vi "IMAQDevice.destructor.vi"(0 "i ref in":refnum<vi>, 5 "error in (no error)":errorcluster) -> (19 "error out":errorcluster)   [LabVIEW 2014, in "IMAQDevice.lvlib"]
doc: "This is the destructor of a class.\n\nLicense Agreement for this software:\n\nCopyright (C)\nGesellschaft für Schwerionenforschung, GSI\nPlanckstr. 1\n64291 Darmstadt\nGermany\n\nContact: D.Beck@gsi.de \n\nThis program is free software; you can redistribute it and/or modify it under the terms of the \nGNU General Public License as published by the Free Software Foundation; either version 2 of \nthe license, or (at your option) any later version.\n\nThis program is distributed in the hope that it will be useful, but WITHOUT ANY WARRANTY; \nwithout even the implied warranty of MERCHANTABILITY or FITNESS FOR A PARTICULAR PURPOSE. See the GNU General License for more details (http://www.gnu.org).\n\nGesellschaft für Schwerionenforschung, GSI\nPlanckstr. 1, 64291 Darmstadt, Germany\nFor all questions and ideas contact: M.Richter@gsi.de, H.Brand@gsi.de or D.Beck@gsi.de.\nLast update: 16-JUN-2004"
uses:
  IMAQDevice.lvlib
  CSCore/CSApplicationBaseClasses/DeviceBase/DeviceBase.lvlib
  CSlibraries-extern/HGF/HGF_LVC/HGF_BaseClasses/HGF_Factory/HGF_Factory.lvclass
  CSlibraries-extern/DimLVEvent/LVDimInterface/LVDimInterface.lvlib
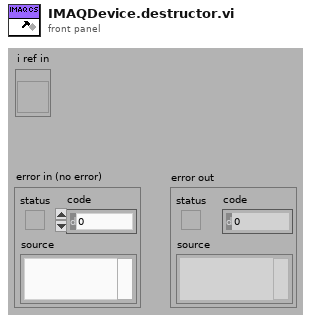
[diagram p1: front panel]
types:
  T1 = typedef "IMAQDevice.lvlib/IMAQDevice.i attribute.ctl" = cluster{"HGF_IMAQ.lvlib:HGF_IMAQDevice.lvclass":refnum<class "HGF_IMAQDevice.lvclass">, "Image":T2, "TimeStampID":i32, "Image IDs":i32[], "NumberOfImagesID":i32, "JPEG?":bool, "JPEGID":i32, "JPEG_ImageID":i32, "TriggerModeID":i32, "OffsetFromLeft":i32, "OffsetFromTop":i32, "HorizontalPixelPerMm":dbl, "VerticalPixelPerMm":dbl, "Grid":cluster{"1":cluster{i32, i32}, "2":cluster{i32, i32}, "3":cluster{i32, i32}, "4":cluster{i32, i32}}, "GridR":cluster{"1":cluster{dbl, dbl}, "2":cluster{dbl, dbl}, "3":cluster{dbl, dbl}, "4":cluster{dbl, dbl}}, "CameraTypeID":i32, "CameraInfos":cluster{"Camera Name-Array":string[], "own Camera Type":string}, "TakeMeasurement?":bool, "TriggerArmedID":i32, "Mirroring":i16, "Rotation":dbl}
  T2 = typedef "IMAQ Image.ctl" = refnum<image>
  T3 = enum16{"SetAttribute", "GetAttribute", "CreateAttribute", "DestroyAttribute", "DestroyAllAtributes"}
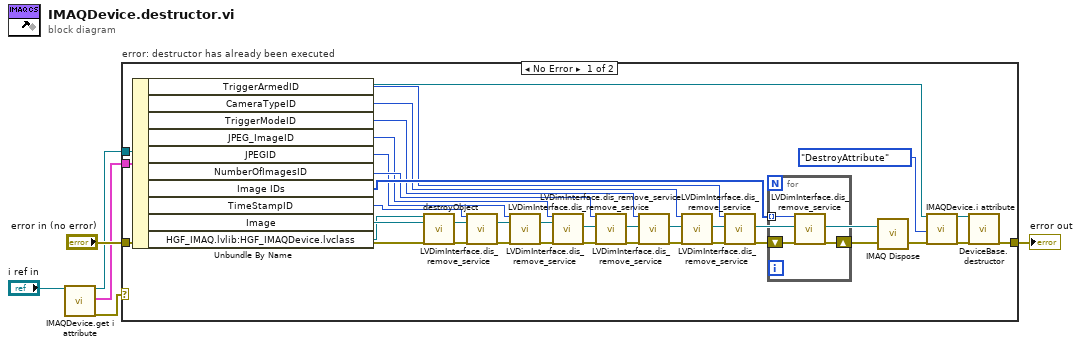
[diagram p0: block diagram]
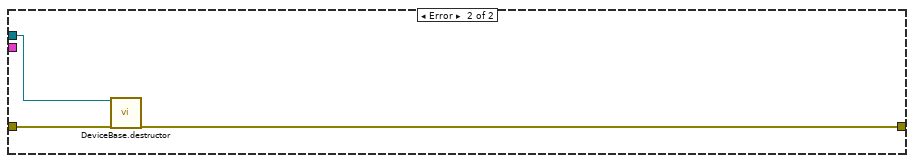
[diagram p2: hidden frame]
diagram:
  n1 = call "IMAQDevice.get i attribute.vi"("i ref in"="i ref in") -> ("i ref out"=w2:refnum<vi>, "i attribute"=w1:T1, "error out"=w3:errorcluster)  [unwired: 16 in]
  n2 = case "error: destructor has already been executed" shown="No Error" w3 {
    tunnel: [w19 w37] -> w6
    tunnel: "error in (no error)" -> [w26 w38]
    tunnel: w2 -> [w30 w39]
    tunnel: w1 -> [w29 _]
    frame No Error {
      n3 = Unbundle By Name(w29) -> ("TriggerArmedID"=w7:i32, "CameraTypeID"=w10:i32, "TriggerModeID"=w12:i32, "JPEG_ImageID"=w14:i32, "JPEGID"=w17:i32, "NumberOfImagesID"=w20:i32, "Image IDs"=w21:i32[], "TimeStampID"=w24:i32, "Image"=w27:T2, "HGF_IMAQ.lvlib:HGF_IMAQDevice.lvclass"=w25:refnum<class "HGF_IMAQDevice.lvclass">)
      n4 = call "destroyObject.vi"("HGF_Factory"=w25, "error in (no error)"=w26) -> ("error out"=w23:errorcluster)  [unwired: 17 in]
      n5 = call "LVDimInterface.dis_remove_service.vi"("my_serviceID"=w24, "error in (no error)"=w23) -> ("error out"=w18:errorcluster)  [unwired: 17 in]
      n6 = call "LVDimInterface.dis_remove_service.vi"("my_serviceID"=w17, "error in (no error)"=w18) -> ("error out"=w16:errorcluster)  [unwired: 17 in]
      n7 = call "LVDimInterface.dis_remove_service.vi"("my_serviceID"=w14, "error in (no error)"=w16) -> ("error out"=w15:errorcluster)  [unwired: 17 in]
      n8 = call "LVDimInterface.dis_remove_service.vi"("my_serviceID"=w20, "error in (no error)"=w15) -> ("error out"=w13:errorcluster)  [unwired: 17 in]
      n9 = call "LVDimInterface.dis_remove_service.vi"("my_serviceID"=w12, "error in (no error)"=w13) -> ("error out"=w11:errorcluster)  [unwired: 17 in]
      n10 = call "LVDimInterface.dis_remove_service.vi"("my_serviceID"=w10, "error in (no error)"=w11) -> ("error out"=w9:errorcluster)  [unwired: 17 in]
      n11 = call "LVDimInterface.dis_remove_service.vi"("my_serviceID"=w7, "error in (no error)"=w9) -> ("error out"=w8:errorcluster)  [unwired: 17 in]
      n12 = for {
        shift-right: [w35] -> w22
        shift-left: w8 -> [w36]
        tunnel: w21 -> [w34] mode=indexing
        n13 = call "LVDimInterface.dis_remove_service.vi"("my_serviceID"=w34, "error in (no error)"=w36) -> ("error out"=w35:errorcluster)  [unwired: 17 in]
      }
      n14 = call "IMAQ Dispose"("Image"=w27, "error in (no error)"=w22) -> ("error out"=w28:errorcluster)  [unwired: 1 in, 3 out]
      n15 = call "IMAQDevice.i attribute.vi"("VI Refnum"=w30, "Action"=T3."DestroyAttribute", "error in (no error)"=w28) -> ("VI Refnum out"=w32:refnum<vi>, "error out"=w31:errorcluster)  [unwired: 14 in, 1 out]
      n16 = call "DeviceBase.destructor.vi"("i ref in"=w32, "error in (no error)"=w31) -> ("error out"=w19:errorcluster)  [unwired: 17 in]
    }
    frame Error {
      n17 = call "DeviceBase.destructor.vi"("i ref in"=w39, "error in (no error)"=w38) -> ("error out"=w37:errorcluster)  [unwired: 17 in]
    }
  }
  "error out" <- w6
